vi "Levelmeter_Check_Queue.vi"(7 "error in (no error)":errorcluster, 10 "queue":refnum<queue>) -> (0 "error out":errorcluster, 1 "Mischer Levelmeter  Control":T1={"N-Shield Refill"=FALSE, "Automatic Refill Shield"=TRUE, "Trap Refill"=FALSE, "Automatic Refill Trap"=TRUE}, 3 "New Entries?":bool)   [LabVIEW 2019]
uses:
  Mischer/Mischer_Levelmeter_Control.ctl
panel:
  out "Numeric":i32
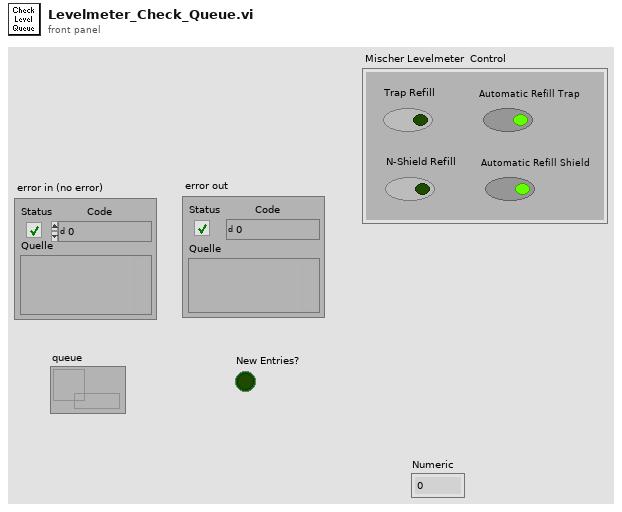
[diagram p1: front panel]
types:
  T1 = typedef "Mischer_Levelmeter_Control.ctl" = cluster{"N-Shield Refill":bool, "Automatic Refill Shield":bool, "Trap Refill":bool, "Automatic Refill Trap":bool}
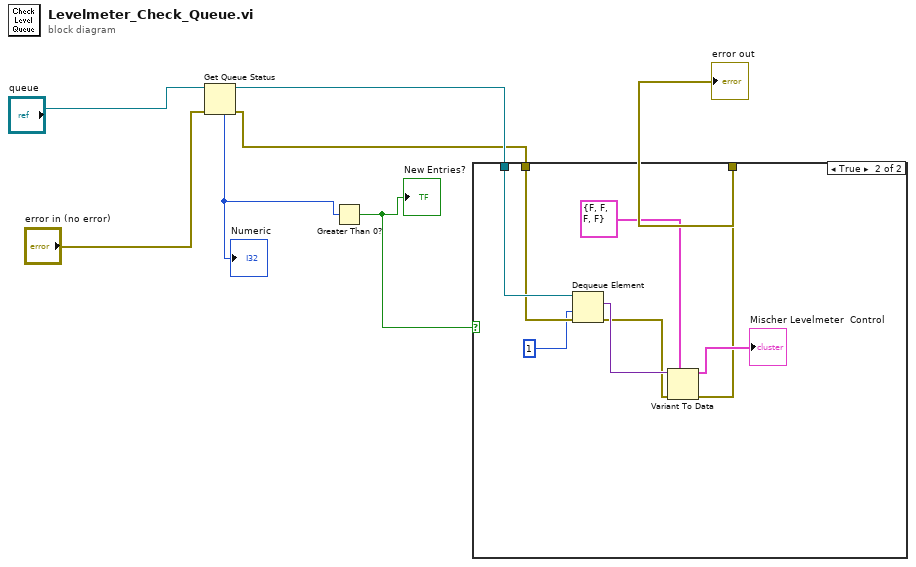
[diagram p0: block diagram]
diagram:
  n1 = Get Queue Status(queue="queue", error in (no error)="error in (no error)") -> (queue out=w3:refnum<queue>, error out=w2:errorcluster, # elements in queue=w5:i32)  [unwired: 1 in, 5 out]
  "Numeric" <- w5
  n2 = Greater Than 0?(x=w5) -> (x > 0?=w4:bool)
  "New Entries?" <- w4
  n3 = case shown="True" w4 {
    tunnel: w3 -> [_ w16]
    tunnel: w2 -> [w8 w15]
    tunnel: [w8 w9] -> w1
    frame False {
    }
    frame True {
      n4 = Dequeue Element(queue=w16, timeout in ms (-1)=1, error in (no error)=w15) -> (element=w13:variant, error out=w12:errorcluster)  [unwired: 2 out]
      n5 = Variant To Data(error in=w12, type=T1 {"N-Shield Refill"=FALSE, "Automatic Refill Shield"=FALSE, "Trap Refill"=FALSE, "Automatic Refill Trap"=FALSE} ("Mischer Levelmeter  Control 2"), Variant=w13) -> (data=→"Mischer Levelmeter  Control":T1, error out=w9:errorcluster)
    }
  }
  "error out" <- w1
